vi "Find Command Names.vi"(10 "project root path":path, 11 "TargetItem in":refnum<vi>) -> (2 "Paths":path[](array[path]), 3 "Command Info":T2(array[cluster]))   [LabVIEW 2023]
uses:
  <vilib>/picture/picture.llb/imagedata.ctl
  <vilib>/Utility/Data Type/NI_Data Type.lvlib
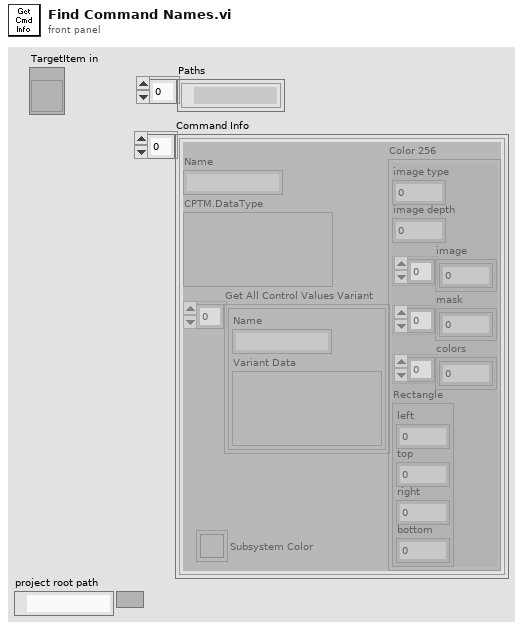
[diagram p1: front panel]
types:
  T1 = typedef "imagedata.ctl" = cluster{"image type":i32, "image depth":i32, "image":u8[], "mask":u8[], "colors":u32[], "Rectangle":cluster{"left":i16, "top":i16, "right":i16, "bottom":i16}}
  T2 = cluster{"Name":string, "CPTM.DataType":variant, "Get All Control Values Variant":cluster{"Name":string, "Variant Data":variant}[], "Color 256":T1, "Subsystem Color":u32}[]
  T3 = typedef "NI_Data Type.lvlib/Type Definition Info.ctl" = cluster{"Name":string, "Timestamp":u32}
  T4 = cluster{"Name":string, "CPTM.DataType":variant, "Get All Control Values Variant":cluster{"Name":string, "Variant Data":variant}[], "ImageData":T1, "Color Box":u32}
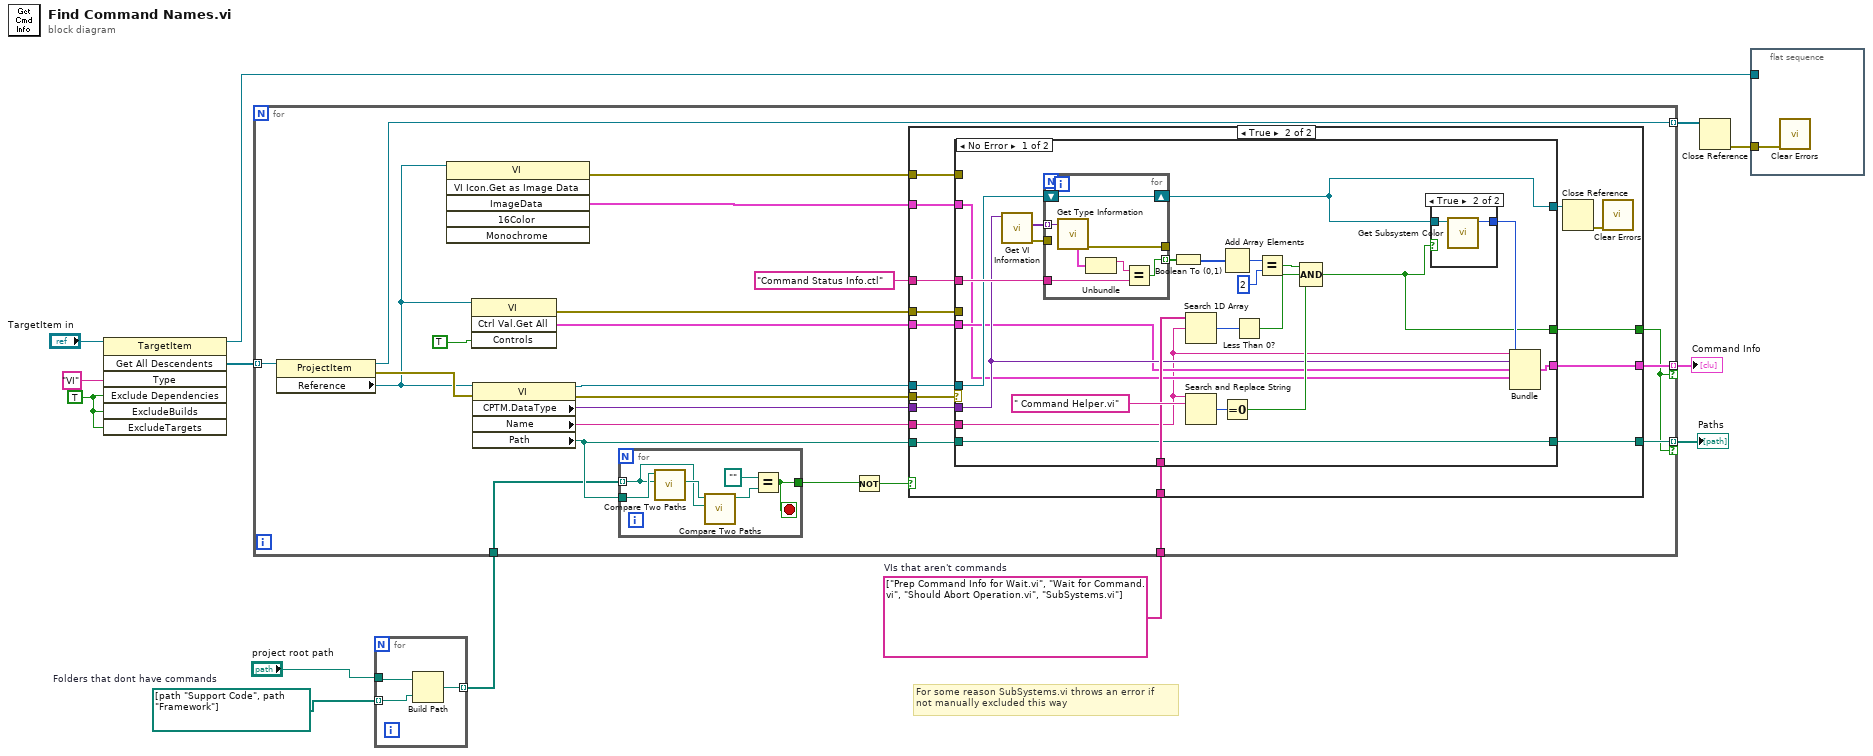
[diagram p0: block diagram]
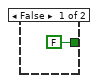
[diagram p2: hidden frame]
diagram:
  w3 = path[] [path "Support Code", path "Framework"]  # Folders that dont have commands
  w10 = TRUE ("ExcludeDependencies")
  w8 = string[] ["Prep Command Info for Wait.vi", "Wait for Command.vi", "Should Abort Operation.vi", "SubSystems.vi"]  # VIs that aren't commands
  # "For some reason SubSystems.vi throws an error if \nnot manually excluded this way"
  n1 = invoke class="TargetItem" method="Get All Descendents"(reference="TargetItem in", "Type"="VI", "Exclude Dependencies"=w10, "ExcludeBuilds"=w10, "ExcludeTargets"=w10) -> (reference out=w4:refnum<vi>, "All Descendents"=w11:refnum<vi>[])  [unwired: 2 in, 5 out]
  n2 = for {
    tunnel: w3 -> [w16] mode=indexing
    tunnel: "project root path" -> [w15]
    tunnel: [w14] -> w1 mode=indexing
    n3 = Build Path(base path=w15, name or relative path=w16) -> (appended path=w14:path)
  }
  n4 = for {
    tunnel: w11 -> [w38] mode=indexing
    tunnel: w8 -> [w36]
    tunnel: [w31] -> w12 mode=indexing if=w21
    tunnel: [w30] -> w13 mode=indexing if=w21
    tunnel: [w23] -> w5 mode=indexing
    tunnel: w1 -> [w19]
    n5 = property class="ProjectItem"(reference=w38) -> (reference out=w23:refnum<vi>, error out=w33:errorcluster, "Reference"=w26:refnum<vi>)  [unwired: 1 in]
    n6 = invoke class="VI" method="VI Icon.Get as Image Data"(reference=w26) -> (error out=w24:errorcluster, "ImageData"=w25:T1)  [unwired: 5 in, 4 out]
    n7 = invoke class="VI" method="Ctrl Val.Get All"(reference=w26, "Controls"=TRUE) -> (error out=w27:errorcluster, "Get All Control Values Variant"=w28:cluster{"Name":string, "Variant Data":variant}[])  [unwired: 2 in, 2 out]
    n8 = property class="VI"(reference=w26, error in=w33) -> (reference out=w22:refnum<vi>, error out=w32:errorcluster, "CPTM.DataType"=w35:variant, "Name"=w34:string, "Path"=w20:path)
    n9 = for {
      tunnel: w19 -> [w93] mode=indexing
      tunnel: w20 -> [w95]
      tunnel: [w90] -> w17
      stop <- w90 stop-if-true
      n10 = call <vilib>:"Compare Two Paths.vi"("Path 2"=w93, "Path 1"=w95) -> ("Common Path"=w94:path)  [unwired: 6 in, 3 out]
      n11 = call <vilib>:"Compare Two Paths.vi"("Path 2"=w93, "Path 1"=w94) -> ("Relative Path from 1 to 2"=w92:path)  [unwired: 6 in, 3 out]
      n12 = Equal?(x=path "", y=w92) -> (x = y?=w90:bool)
    }
    n13 = Not(x=w17) -> (.not. x?=w18:bool)
    n14 = case shown="True" w18 {
      tunnel: "Command Status Info.ctl" ("Name") -> [_ w55]
      tunnel: w36 -> [_ w54]
      tunnel: w35 -> [_ w53]
      tunnel: w34 -> [_ w52]
      tunnel: w32 -> [_ w49]
      tunnel: [_ w48] -> w31
      tunnel: [_ w47] -> w30
      tunnel: w28 -> [_ w46]
      tunnel: w27 -> [_ w45]
      tunnel: w25 -> [_ w44]
      tunnel: w24 -> [_ w43]
      tunnel: w22 -> [_ w42]
      tunnel: [FALSE w41] -> w21
      tunnel: w20 -> [_ w40]
      frame False {
      }
      frame True {
        n15 = case shown="No Error" w49 {
          tunnel: w55 -> [w68 _]
          tunnel: w54 -> [w67 _]
          tunnel: w53 -> [w62 _]
          tunnel: w52 -> [w57 _]
          tunnel: [w59 w89] -> w50
          tunnel: w42 -> [w65 w89]
          tunnel: [w63 _] -> w48
          tunnel: w40 -> [w64 _]
          tunnel: [w64 _] -> w47
          tunnel: w46 -> [w61 _]
          tunnel: w45 -> [_ _]
          tunnel: w44 -> [w60 _]
          tunnel: w43 -> [_ _]
          tunnel: [w56 _] -> w41
          frame No Error {
            n16 = call <vilib>:"Get VI Information.vi"("variant"=w62) -> ("error out"=w71:errorcluster, "VI terminal types"=w70:variant[])  [unwired: 7 in, 2 out]
            n17 = for {
              tunnel: w68 -> [w88]
              tunnel: [w87] -> w69 mode=indexing
              tunnel: w70 -> [w85] mode=indexing
              tunnel: w71 -> [_]
              tunnel: [w84] -> _
              shift-right: [w86] -> w59
              shift-left: w65 -> [w86]
              n18 = call <vilib>:"Get Type Information.vi"("variant"=w85) -> ("error out"=w84:errorcluster, "type definition info"=w83:T3)  [unwired: 6 in, 3 out]
              n19 = Unbundle(w83) -> ("Name"=w82:string)  [unwired: 1 out]
              n20 = Equal?(x=w82, y=w88) -> (x = y?=w87:bool)
            }
            n21 = Boolean To (0,1)(Boolean=w69) -> (0, 1=w66:i16[])
            n22 = Search 1D Array(1D array=w67, element=w57) -> (index of element=w74:i32)  [unwired: 1 in]
            n23 = Search and Replace String(input string=w57, search string=" Command Helper.vi") -> (number of replacements=w76:i32)  [unwired: 6 in, 3 out]
            n24 = Add Array Elements(numeric array=w66) -> (sum=w78:i16)
            n25 = Equal To 0?(x=w76) -> (x = 0?=w77:bool)
            n26 = Less Than 0?(x=w74) -> (x < 0?=w75:bool)
            n27 = Equal?(x=w78, y=2) -> (x = y?=w79:bool)
            n28 = Compound Arithmetic op=AND(w79, w75, w77) -> (w56:bool)
            n29 = case shown="True" w56 {
              tunnel: w59 -> [_ w81]
              tunnel: [_ w80] -> w58
              frame False {
              }
              frame True {
                n30 = call "Get Subsystem Color.vi"("VI in"=w81) -> ("Color Box"=w80:u32)  [unwired: 10 in]
              }
            }
            n31 = Bundle("Name"=w57, "CPTM.DataType"=w62, "Get All Control Values Variant"=w61, "ImageData"=w60, "Color Box"=w58) -> (w63:T4)  [unwired: 1 in]
          }
          frame Error {
          }
        }
        n32 = Close Reference(reference=w50) -> (error out=w51:errorcluster)  [unwired: 1 in]
        n33 = call <vilib>:"Clear Errors.vi"("error in (no error)"=w51) -> ()  [unwired: 5 in, 2 out]
      }
    }
  }
  "Paths" <- w13
  "Command Info" <- w12
  n34 = Close Reference(reference=w5) -> (error out=w6:errorcluster)  [unwired: 1 in]
  n35 = flat-sequence {
    tunnel: w6 -> [w96]
    tunnel: w4 -> [_]
    frame #0 {
      n36 = call <vilib>:"Clear Errors.vi"("error in (no error)"=w96) -> ()  [unwired: 5 in, 2 out]
    }
  }
